vi "Probability Array.vi"(7 "QuWire in":refnum<class "QuWire.lvclass">) -> ()   [LabVIEW 2020]
uses:
  QuSim/QuWire/QuWire.lvclass
panel:
  out "Qubit Count":i32
  out "Basis States and Probabilities":cluster{"State":i32, "Probability":dbl}[](array[cluster]) {"Probability" format="%#.6f"; "State" format="%07b"}
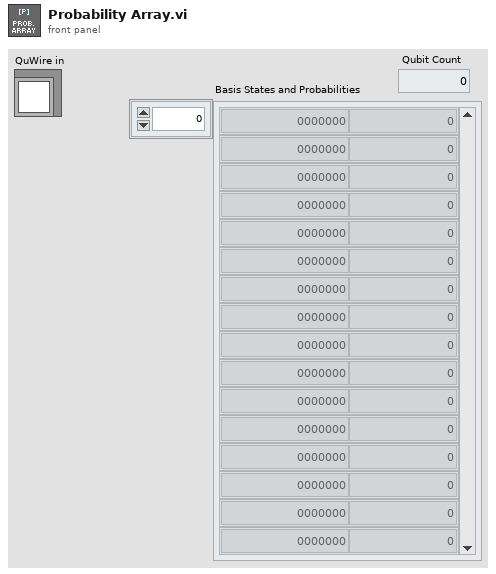
[diagram p1: front panel]
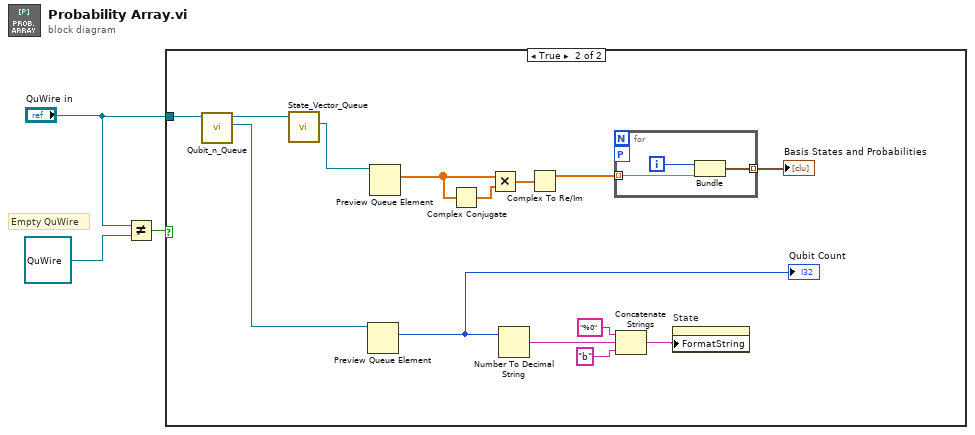
[diagram p0: block diagram]
diagram:
  # "Empty QuWire"
  n1 = Not Equal?(x="QuWire in", y=refnum<class "QuWire.lvclass"> refnum ("QuWire in")) -> (x != y?=w2:bool)
  n2 = case shown="True" w2 {
    tunnel: "QuWire in" -> [_ w12]
    frame False {
    }
    frame True {
      n3 = call "Qubit_n_Queue.vi"("QuWire in"=w12) -> ("Qubit n"=w11:refnum<queue>, "QuWire out"=w13:refnum<class "QuWire.lvclass">)  [unwired: 8 in, 1 out]
      n4 = call "State_Vector_Queue.vi"("QuWire in"=w13) -> ("State Vector Queue"=w17:refnum<queue>)  [unwired: 8 in, 2 out]
      n5 = Preview Queue Element(queue=w11) -> (element=w6:i32)  [unwired: 2 in, 3 out]
      "Qubit Count" <- w6
      n6 = Preview Queue Element(queue=w17) -> (element=w15:cdb[])  [unwired: 2 in, 3 out]
      n7 = Complex Conjugate(1:w15) -> (0:w16:cdb[])
      n8 = Multiply(x=w15, y=w16) -> (x*y=w14:cdb[])
      n9 = Number To Decimal String(number=w6) -> (decimal integer string=w7:string)  [unwired: 1 in]
      n10 = Complex To Re/Im(x + iy=w14) -> (x=w4:dbl[])  [unwired: 1 out]
      n11 = for {
        tunnel: w4 -> [w19] mode=indexing
        tunnel: [w18] -> w10 mode=indexing
        workers-P: _ -> [_]
        i -> [w20]
        n12 = Bundle(w20, "Complex Matrix Element"=w19) -> (w18:cluster{i32, "Complex Matrix Element":dbl})  [unwired: 1 in]
      }
      "Basis States and Probabilities" <- w10
      n13 = Concatenate Strings("%0" ("string"), w7, "b" ("string")) -> (w5:string)
      n14 = property on="State" class="DigNum (strict)"("FormatString"=w5) -> ()  [unwired: 2 in, 2 out]
    }
  }
